vi "ImageSaveImage-2D.vi"(6 "Modify Min Max":bool, 8 "error in (no error)":errorcluster, 9 "Maxs":dbl[](array[numeric]), 10 "Mins":dbl[](array[numeric]), 11 "Image in":refnum<class "Image.lvclass">) -> (0 "error out":errorcluster, 3 "Image out":refnum<class "Image.lvclass">)   [LabVIEW 2012, in "Image.lvclass"]
uses:
  classes/Image.lvclass
  classes/Image.lvclass/Image.ctl
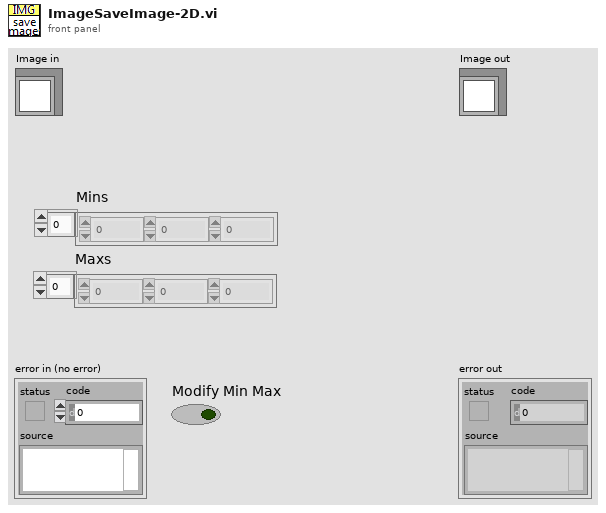
[diagram p1: front panel]
types:
  T1 = typedef "ScanMode.ctl" = enum16{"None", "Continuous", "Point Scan (CH3 cursor)", "Point Scan Move (CH3 cursor)", "Grab", "Grab Move Stage", "Grab Move Z-stage", "Cont. Move Z-stage", "Spec Move Stage", "Spec Move Cont", "Surf Calib"}
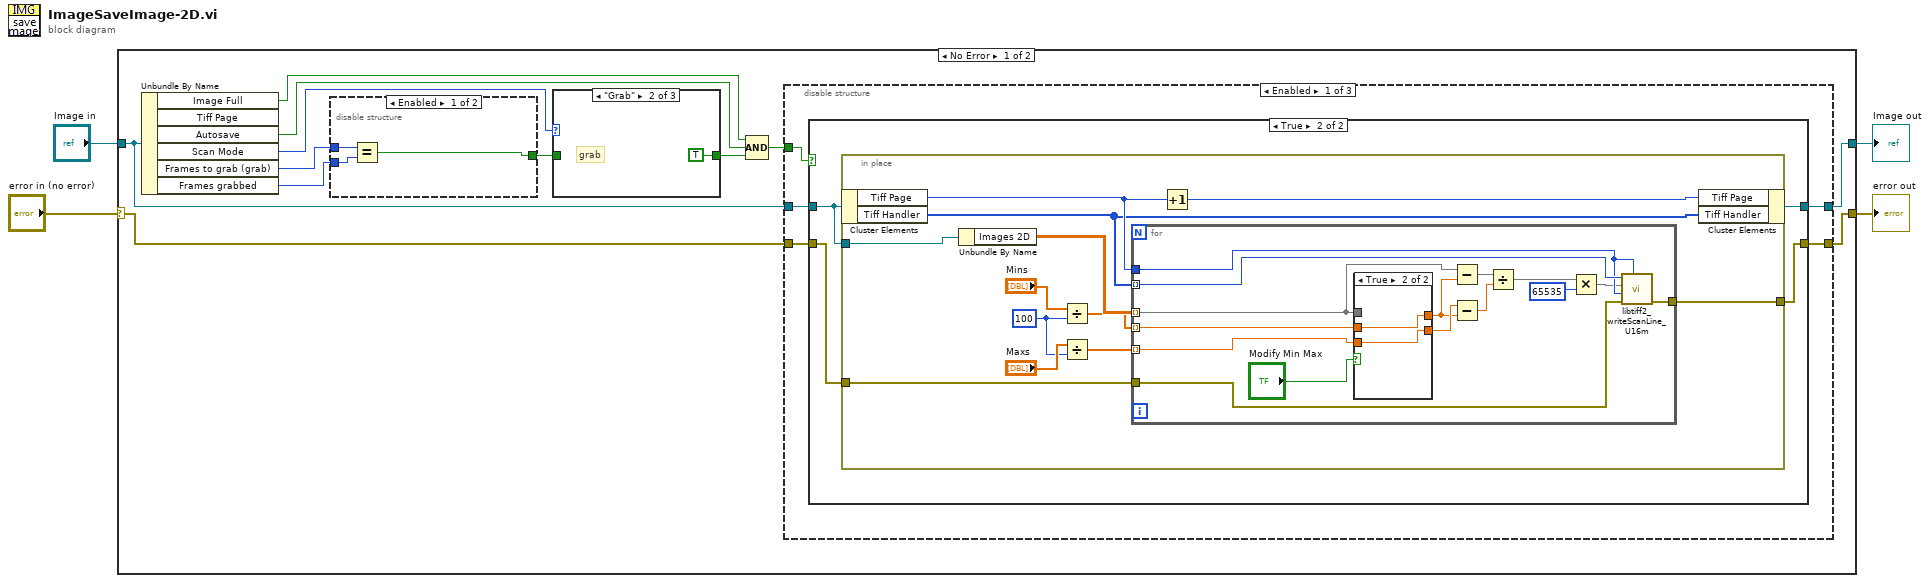
[diagram p0: block diagram]
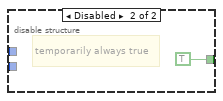
[diagram p2: hidden frame]
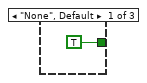
[diagram p3: hidden frame]
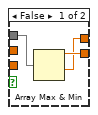
[diagram p6: hidden frame]
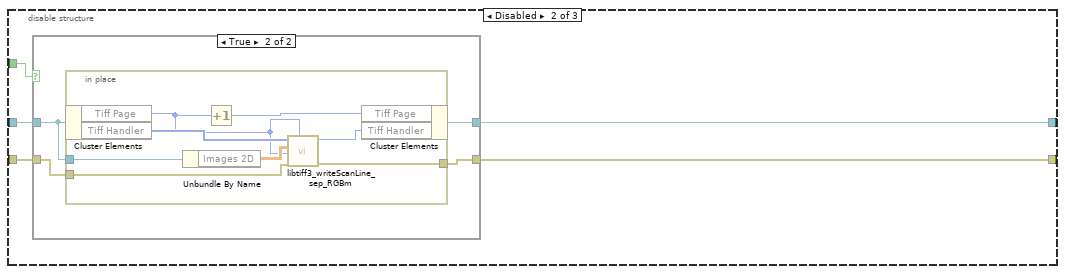
[diagram p7: hidden frame]
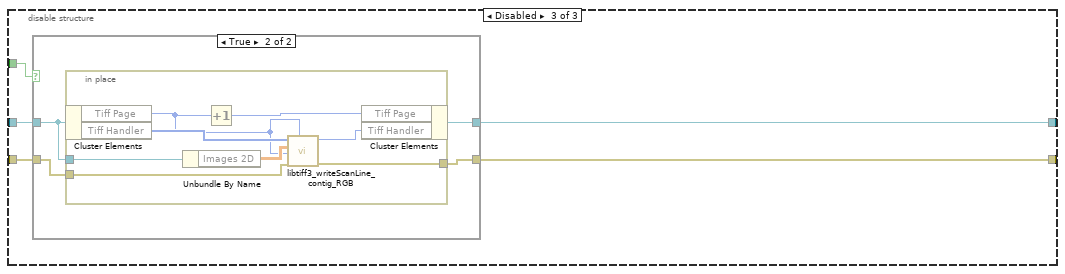
[diagram p9: hidden frame]
diagram:
  n1 = case shown="No Error" "error in (no error)" {
    selector: "error in (no error)" -> [w16 w106]
    tunnel: [w15 w106] -> w3
    tunnel: [w13 w105] -> w2
    tunnel: "Image in" -> [w14 w105]
    frame No Error {
      n2 = Unbundle By Name(w14) -> ("Image Full"=w5:bool, "Autosave"=w10:bool, "Scan Mode"=w8:T1, "Frames to grab (grab)"=w12:i32, "Frames grabbed"=w11:i32)  [unwired: 1 out]
      n3 = disable-structure shown="Enabled" {
        disable-tunnel: w12 -> [w19 _]
        disable-tunnel: w11 -> [w18 _]
        disable-tunnel: [w17 TRUE] -> w7
        frame Enabled {
          n4 = Equal?(x=w19, y=w18) -> (x = y?=w17:bool)
        }
        frame Disabled {
          # "temporarily always true"
        }
      }
      n5 = case shown="\"Grab\"" w8 {
        tunnel: w7 -> [_ _ w23]
        tunnel: [TRUE TRUE w23] -> w6
        frame "None", Default {
        }
        frame "Grab" {
          # "grab"
        }
        frame "Grab Move Stage" {
          # "grab movestage"
        }
      }
      n6 = Compound Arithmetic op=AND(w5, w10, w6) -> (w9:bool)
      n7 = disable-structure shown="Enabled" {
        disable-tunnel: w16 -> [w28 w71 w90]
        disable-tunnel: [w27 w70 w89] -> w15
        disable-tunnel: w14 -> [w26 w69 w88]
        disable-tunnel: [w25 w68 w87] -> w13
        disable-tunnel: w9 -> [w24 w67 w86]
        frame Enabled {
          n8 = case shown="True" w24 {
            tunnel: w28 -> [w29 w34]
            tunnel: [w29 w33] -> w27
            tunnel: w26 -> [w30 w32]
            tunnel: [w30 w31] -> w25
            frame False {
            }
            frame True {
              n9 = in-place {
                in-place-border: w34 -> [w43]
                in-place-border: [w42] -> w33
                in-place-border: w32 -> [w45]
                w37 = 100
                n10 = in-place-cluster #1(w32) -> ("Tiff Page"=w44:u32, "Tiff Handler"=w40:u32[])
                n11 = Unbundle By Name(w45) -> ("Images 2D"=w41:dbl[][][])
                n12 = Divide(x="Mins", y=w37) -> (x/y=w36:dbl[])
                n13 = Divide(x="Maxs", y=w37) -> (x/y=w35:dbl[])
                n14 = for {
                  tunnel: w40 -> [w61] mode=indexing
                  tunnel: w44 -> [w60]
                  tunnel: w43 -> [w59]
                  tunnel: [w58] -> w42
                  tunnel: w41 -> [w52] mode=indexing
                  tunnel: w36 -> [w48] mode=indexing
                  tunnel: w35 -> [w49] mode=indexing
                  n15 = case shown="True" "Modify Min Max" {
                    tunnel: w52 -> [w64 _]
                    tunnel: [w63 w66] -> w51
                    tunnel: [w62 w65] -> w50
                    tunnel: w49 -> [_ w66]
                    tunnel: w48 -> [_ w65]
                    frame False {
                      n16 = Array Max & Min(array=w64) -> (max value=w63:dbl, min value=w62:dbl)  [unwired: 2 out]
                    }
                    frame True {
                    }
                  }
                  n17 = Subtract(x=w52, y=w50) -> (x-y=w57:dbl[][])
                  n18 = Subtract(x=w51, y=w50) -> (x-y=w56:dbl)
                  n19 = Divide(x=w57, y=w56) -> (x/y=w55:dbl[][])
                  n20 = Multiply(x=w55, y=65535) -> (x*y=w53:dbl[][])
                  n21 = call "libtiff2_writeScanLine_U16m.vi"("totalpages"=w60, "error in (no error)"=w59, "page"=w60, "Data"=w53, "Handle"=w61) -> ("error out"=w58:errorcluster)  [unwired: 5 in, 1 out]
                }
                n22 = Increment(x=w44) -> (x+1=w46:u32)
                n23 = in-place-cluster #1("Tiff Page"=w46, "Tiff Handler"=w40) -> (w31:refnum<class "Image.lvclass">)
              }
            }
          }
        }
        frame Disabled {
          n24 = case shown="True" w67 {
            tunnel: w71 -> [w72 w77]
            tunnel: [w72 w76] -> w70
            tunnel: w69 -> [w73 w75]
            tunnel: [w73 w74] -> w68
            frame False {
            }
            frame True {
              n25 = in-place {
                in-place-border: w77 -> [w83]
                in-place-border: [w82] -> w76
                in-place-border: w75 -> [w84]
                n26 = in-place-cluster #2(w75) -> ("Tiff Page"=w79:u32, "Tiff Handler"=w81:u32[])
                n27 = Unbundle By Name(w84) -> ("Images 2D"=w80:dbl[][][])
                n28 = Increment(x=w79) -> (x+1=w85:u32)
                n29 = call "libtiff3_writeScanLine_sep_RGBm.vi"("totalpages"=w79, "error in (no error)"=w83, "page"=w79, "Data"=w80, "Handle"=w81) -> ("error out"=w82:errorcluster, "Handle out"=w78:i32)  [unwired: 5 in]
                n30 = in-place-cluster #2("Tiff Page"=w85, "Tiff Handler"=w78) -> (w74:refnum<class "Image.lvclass">)
              }
            }
          }
        }
        frame Disabled {
          n31 = case shown="True" w86 {
            tunnel: w90 -> [w91 w96]
            tunnel: [w91 w93] -> w89
            tunnel: w88 -> [w92 w95]
            tunnel: [w92 w94] -> w87
            frame False {
            }
            frame True {
              n32 = in-place {
                in-place-border: w96 -> [w99]
                in-place-border: w95 -> [w103]
                in-place-border: [w97] -> w93
                n33 = in-place-cluster #3(w95) -> ("Tiff Page"=w100:u32, "Tiff Handler"=w102:u32[])
                n34 = Unbundle By Name(w103) -> ("Images 2D"=w101:dbl[][][])
                n35 = Increment(x=w100) -> (x+1=w104:u32)
                n36 = call "libtiff3_writeScanLine_contig_RGB.vi"("totalpages"=w100, "error in (no error)"=w99, "page"=w100, "Data"=w101, "Handle"=w102) -> ("error out"=w97:errorcluster, "Handle out"=w98:i32)  [unwired: 5 in]
                n37 = in-place-cluster #3("Tiff Page"=w104, "Tiff Handler"=w98) -> (w94:refnum<class "Image.lvclass">)
              }
            }
          }
        }
      }
    }
    frame Error {
    }
  }
  "error out" <- w3
  "Image out" <- w2
